vi "Process.vi"(8 "error in (no error)":errorcluster, 11 "RemoteControl":refnum<class "RemoteControl.lvclass">) -> (0 "error out":errorcluster, 3 "RemoteControl out":refnum<class "RemoteControl.lvclass">)   [LabVIEW 2019, in "RemoteControl.lvlib" / "RemoteControl.lvclass"]
doc: "---------------------------------------------------------------\nJKI State Machine Objects™\nhttp://jki.net/state-machine-objects/\nCopyright (C) 2005-2015, JKI <info@jki.net>\nALL RIGHTS RESERVED"
uses:
  RemoteControl.lvclass
  Typedefs/Message--Cluster.ctl
  Typedefs/RC Process Type--Enum.ctl
  <vilib>/ErrorRing/Error Ring.xnode
  <userlib>/LevyLab/Debug/Debug.lvlib
  C:/Program Files (x86)/National Instruments/LabVIEW 2019/vi.lib/JKI/JKI SMO/SMO/SMO.lvclass
  <vilib>/JKI/JKI SMO/SMO/SMO.lvclass
  <vilib>/JKI/JKI SMO/SMO/Typedefs/SMOState --Enum.ctl
  <vilib>/JKI/JKI SMO/SMO/Typedefs/Reserve State--Enum.ctl
  <vilib>/JKI/JKI SMO/SMO/Typedefs/Public Events.ctl
panel:
  out "Process Type":string
  out "Message Out":string
  out "Message In":string
  in  "delay response":bool
  in  "create server error":bool
  in  "create listener error":bool
  out "State History":string
  out "Connections":i32
  in  "Message Timing?":bool
  in  "timeout (ms) [500]":i32=500
  in  "stop":bool
  # "Remote Control"
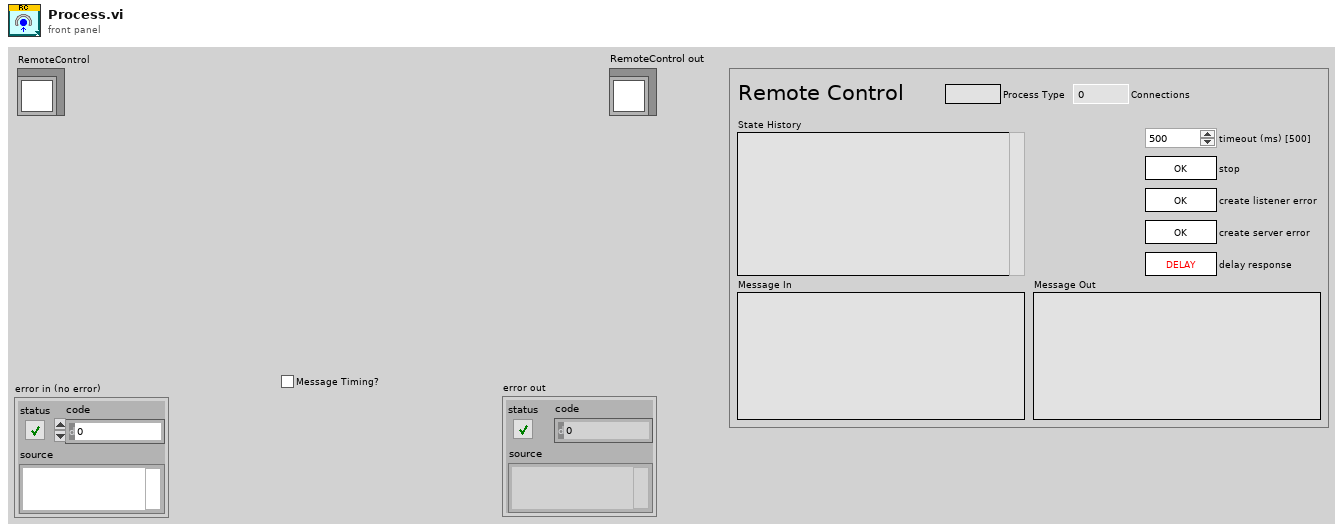
[diagram p1: front panel]
types:
  T1 = enum32{"invalid app kind", "Development System", "Run Time System", "Student Edition", "Embedded LabVIEW", "Evaluation", "Custom"}
  T2 = enum32{"Invalid", "Standard", "Closed", "Hidden", "Minimized", "Maximized"}
  T3 = typedef "RemoteControl.lvlib/RemoteControl.lvclass/Message--Cluster.ctl" = cluster{"Command":string, "Data":variant, "ID":string}
  T4 = typedef "RemoteControl.lvlib/RemoteControl.lvclass/RC Process Type--Enum.ctl" = enum16{"Listener", "Server", "Client"}
  T5 = typedef "RemoteControl.lvclass/Message--Cluster.ctl" = cluster{"Command":string, "Data":variant, "ID":string}
  T6 = typedef "RemoteControl.lvlib/RemoteControl.lvclass/PrivateEvents--RemoteControl.Configure.ctl" = cluster{"address":string, "Port":u16, "AllowedRemote":string, "Commands":string[], "timeout":i32}
  T7 = cluster{"Core":cluster{"Current VI Reference":refnum<vi>, "Close Panel on Exit?":bool, "Last Error":cluster{"error":errorcluster, "previous state":string, "remaining states":string}, "Shutdown?":bool}, "SelfRef":refnum<class "RemoteControl.lvclass">, "Listener":refnum<class "RemoteControl.lvclass">, "RC Process Type":T4, "Configure":T6, "Messages (in)":T3[], "Messages (out)":T3[], "state":enum16{"waiting", "processing"}, "to":i32}
  T8 = cluster{"Current VI Reference":refnum<vi>, "Close Panel on Exit?":bool, "Last Error":cluster{"error":errorcluster, "previous state":string, "remaining states":string}, "Shutdown?":bool}
  T9 = typedef "Debug.lvlib/Attribute.Debug.lvclass/DebugBehavior.ctl" = enum16{"Normal", "Debug"}
  T10 = typedef "SMO.lvclass/Public Events.ctl" = cluster{"Error":refnum<user-event>, "State":refnum<user-event>, "Reserve State":refnum<user-event>}
  T11 = typedef "SMO.lvclass/Protected Events.ctl" = cluster{"StopProcesses":refnum<user-event>, "AbortProcesses":refnum<user-event>, "Config Changed":refnum<user-event>, "Dependency":refnum<user-event>}
  T12 = typedef "RemoteControl.lvlib/RemoteControl.lvclass/PrivateEvents--Cluster.ctl" = cluster{"Configure":refnum<user-event>, "SendMessageToProcess":refnum<user-event>}
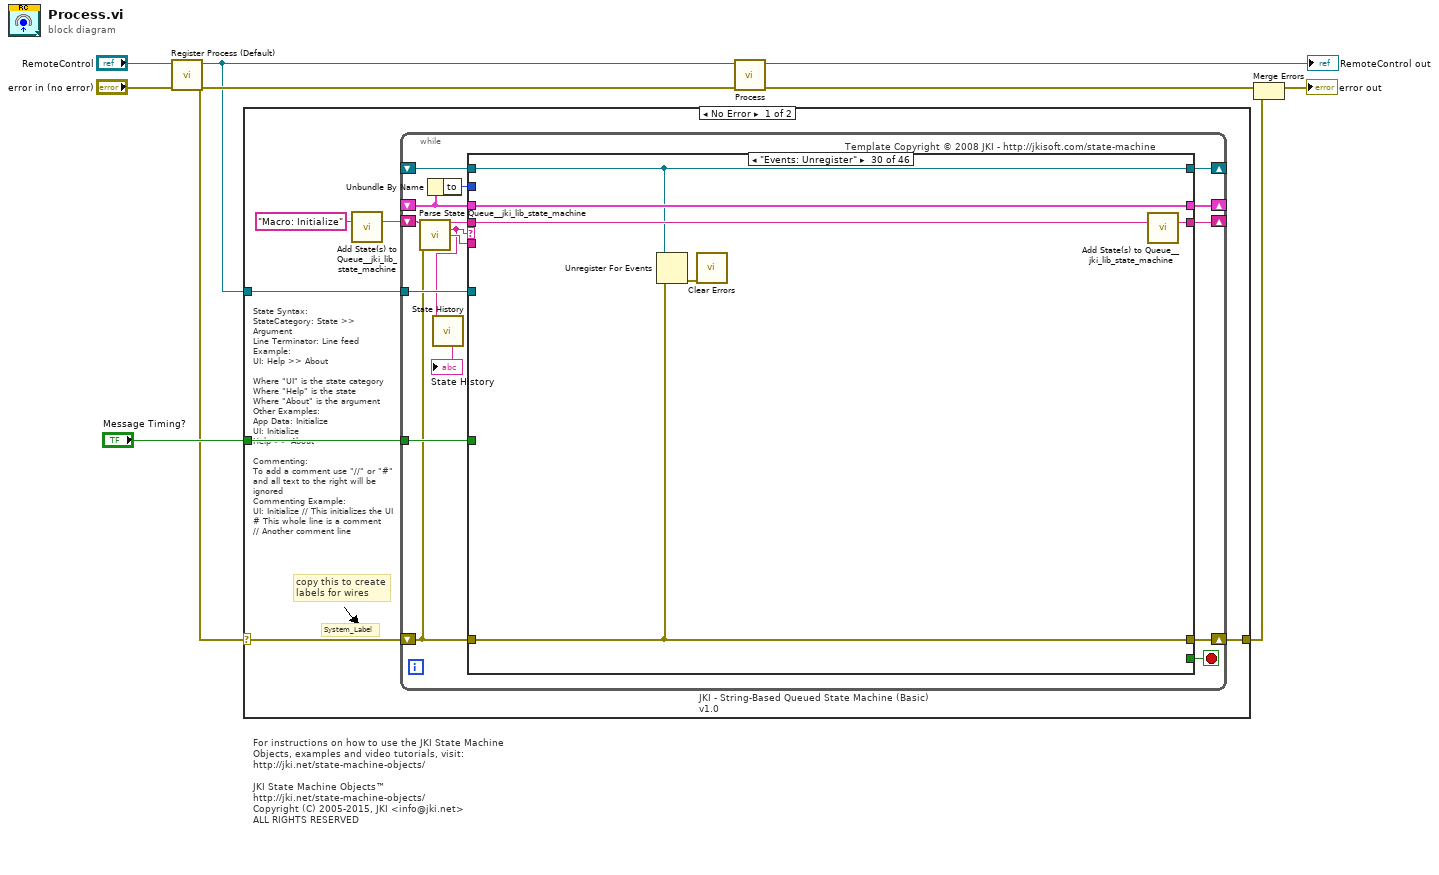
[diagram p0: block diagram]
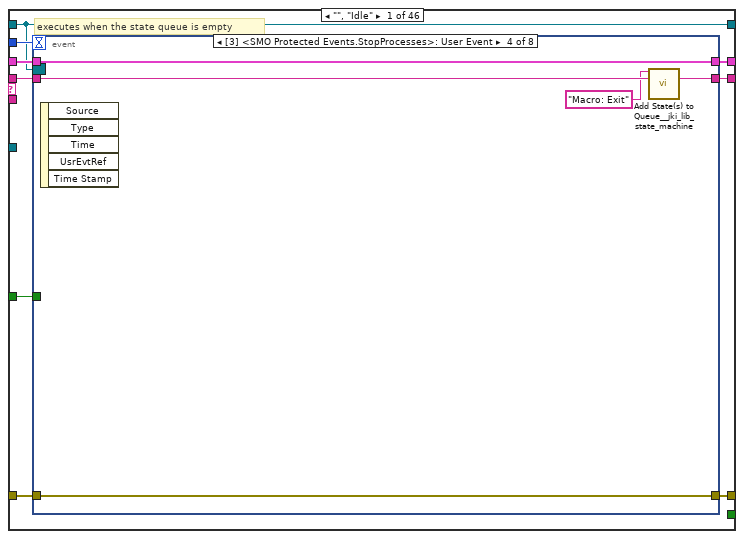
[diagram p2: hidden frame]
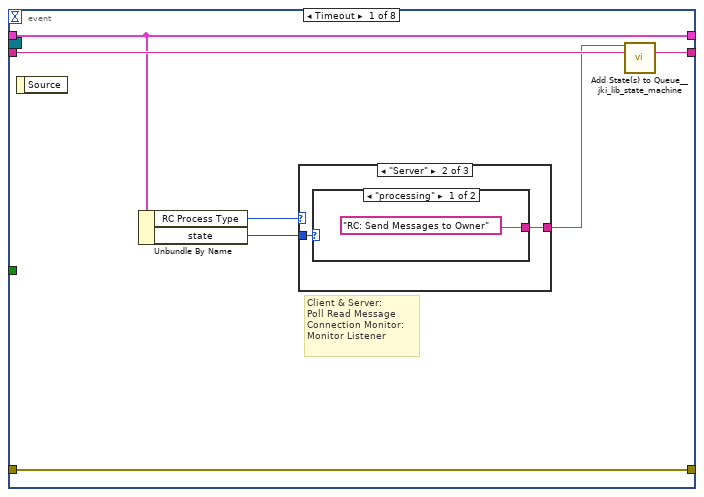
[diagram p3: hidden frame]
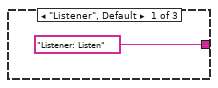
[diagram p4: hidden frame]
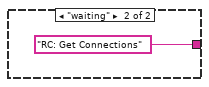
[diagram p5: hidden frame]
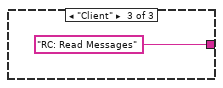
[diagram p6: hidden frame]
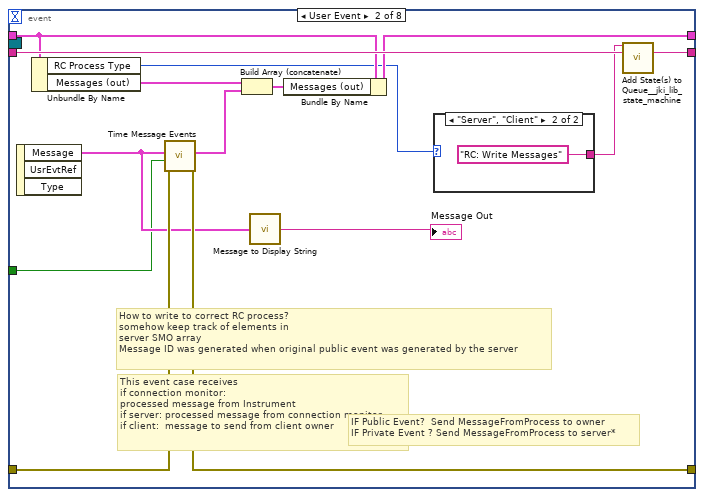
[diagram p7: hidden frame]
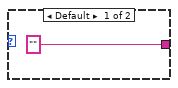
[diagram p8: hidden frame]
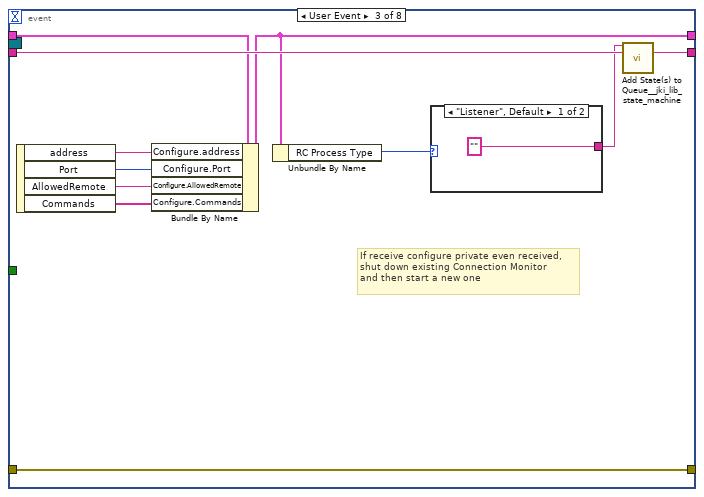
[diagram p9: hidden frame]
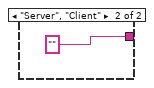
[diagram p10: hidden frame]
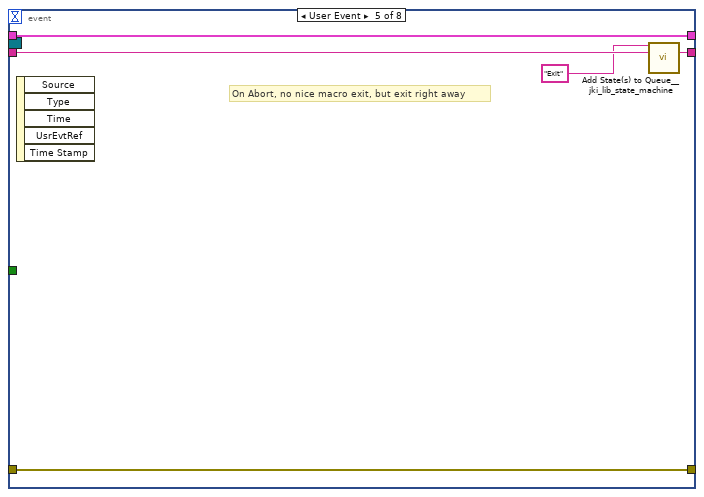
[diagram p11: hidden frame]
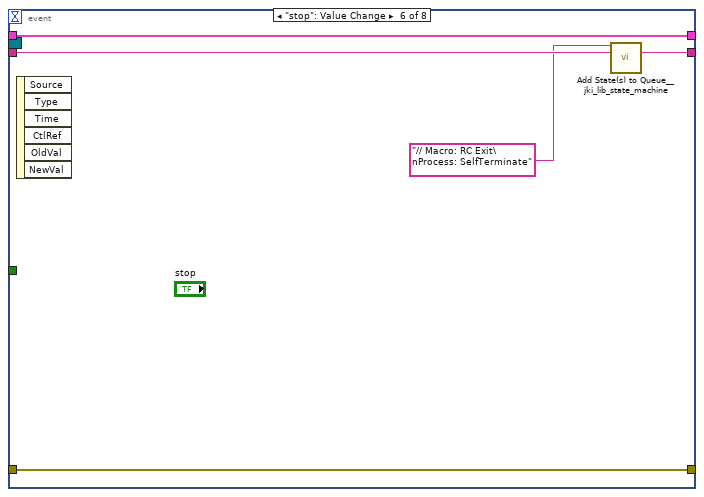
[diagram p12: hidden frame]
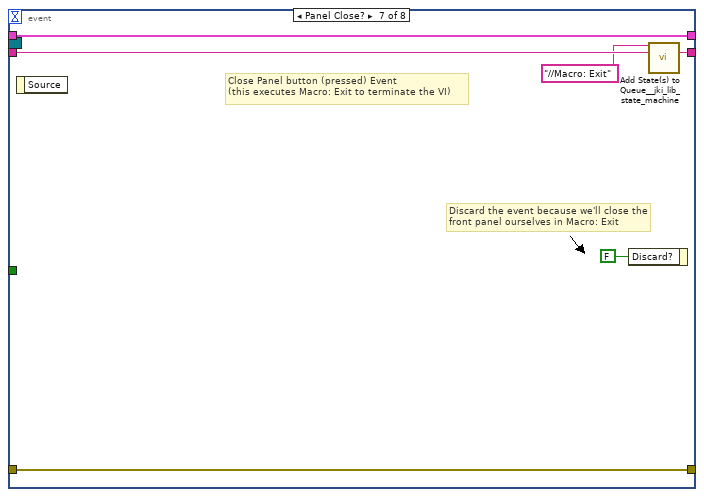
[diagram p13: hidden frame]
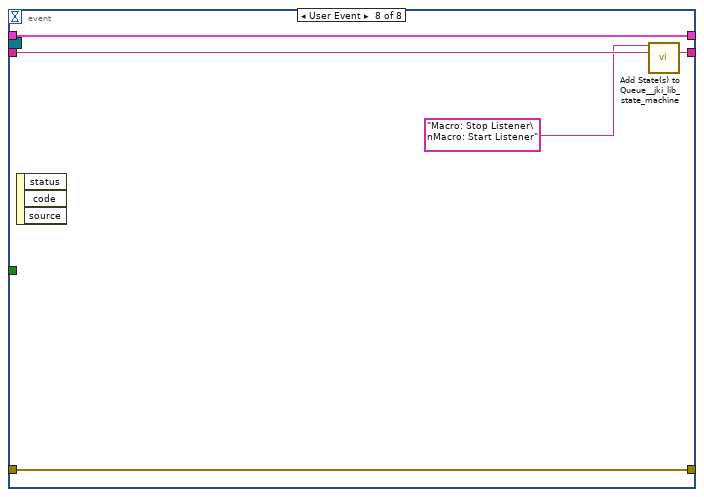
[diagram p14: hidden frame]
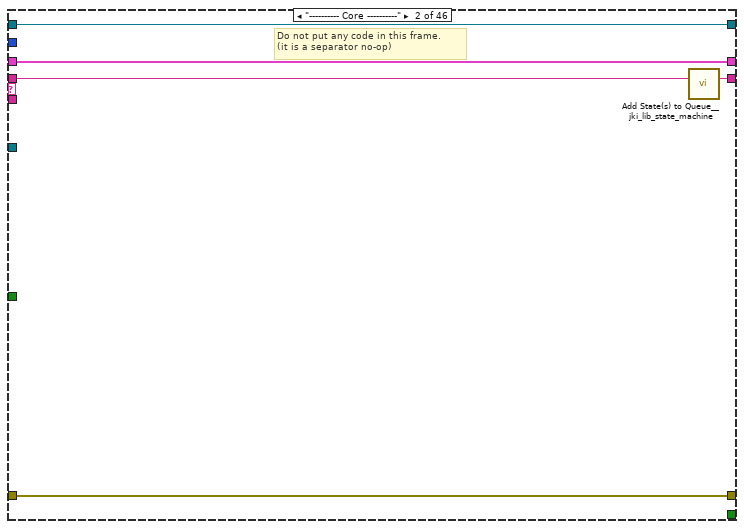
[diagram p15: hidden frame]
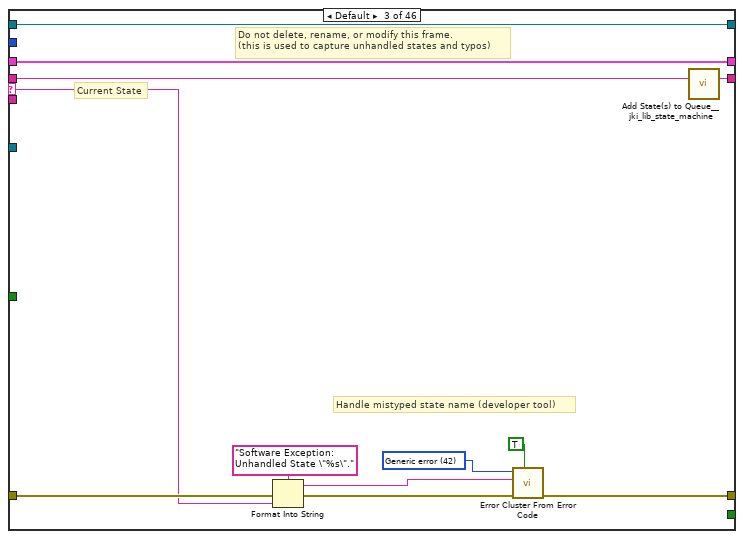
[diagram p16: hidden frame]
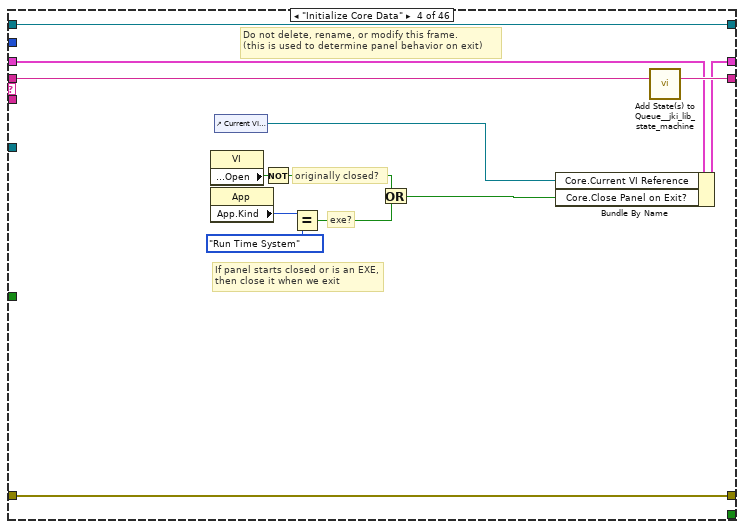
[diagram p17: hidden frame]
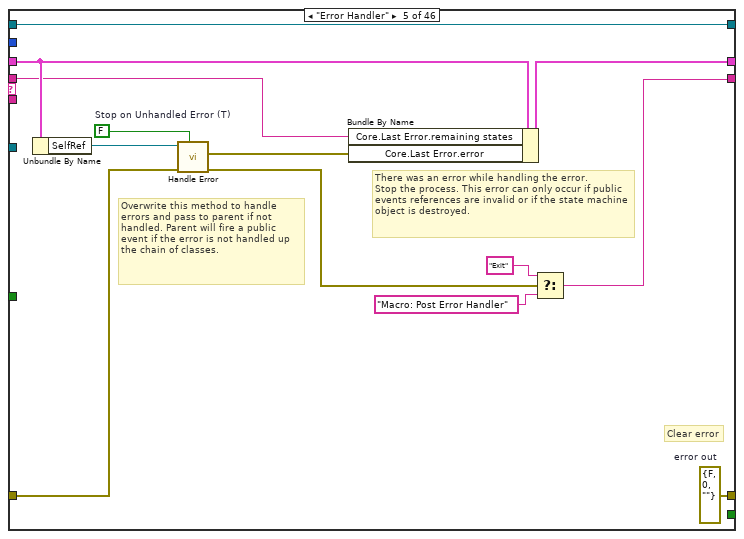
[diagram p18: hidden frame]
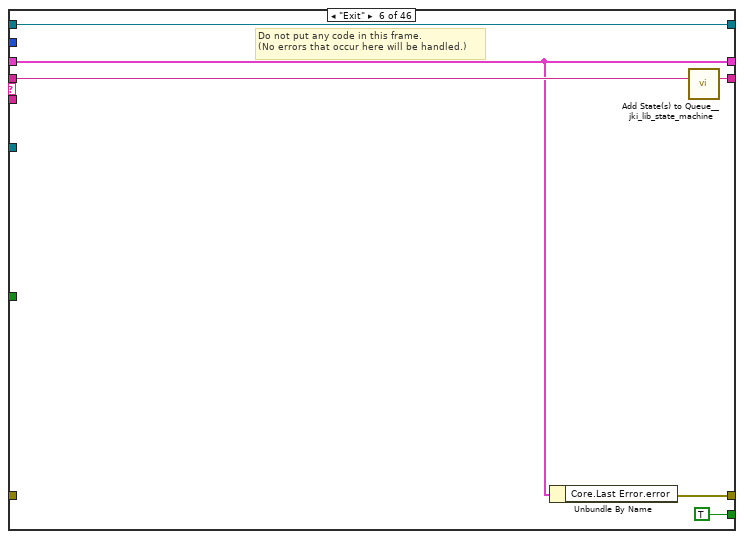
[diagram p19: hidden frame]
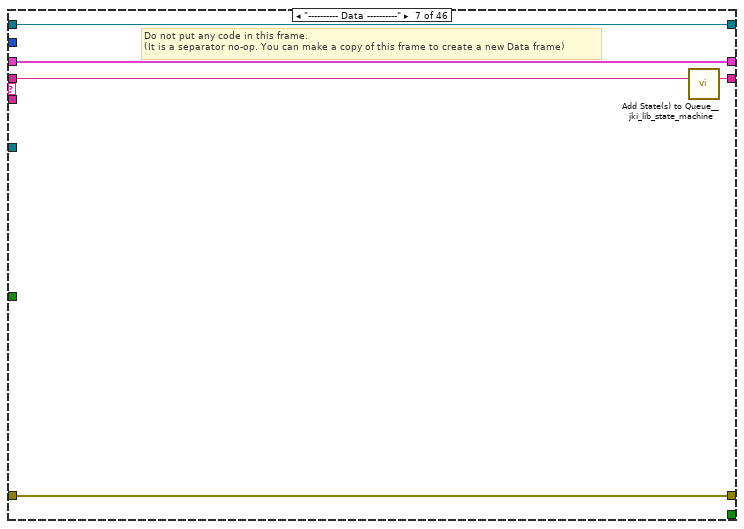
[diagram p20: hidden frame]
diagram:
  # "For instructions on how to use the JKI State Machine Objects, examples and video tutorials, visit:\nhttp://jki.net/state-machine-objects/\n\nJKI State Machine Objects™\nhttp://jki.net/state-machine-objects/\nCopyright (C) 2005-2015, JKI <info@jki.net>\nALL RIGHTS RESERVED"
  n1 = call <vilib>:"Register Process (Default).vi"("error in (no error)"="error in (no error)", "SMO"="RemoteControl") -> ("error out"=w3:errorcluster, "SelfRef"=w2:refnum<class "RemoteControl.lvclass">)  [unwired: 8 in]
  n2 = case shown="No Error" w3 {
    selector: w3 -> [w12 w662]
    tunnel: w2 -> [w13 _]
    tunnel: [w11 w662] -> w5
    tunnel: "Message Timing?" -> [w10 _]
    frame No Error {
      # "State Syntax:\nStateCategory: State >> Argument\nLine Terminator: Line feed\nExample:\nUI: Help >> About\n\nWhere \"UI\" is the state category\nWhere \"Help\" is the state\nWhere \"About\" is the argument\nOther Examples:\nApp Data: Initialize\nUI: Initialize\nHelp >> About\n\nCommenting:\nTo add a comment use \"//\" or \"#\" and all text to the right will be ignored\nCommenting Example:\nUI: Initialize // This initializes the UI\n# This whole line is a comment\n// Another comment line"
      # "copy this to create labels for wires"
      # "System_Label"
      n3 = call <vilib>:"Add State(s) to Queue__jki_lib_state_machine.vi"("State(s) in (\"\")"="Macro: Initialize") -> ("States Out"=w15:string)  [unwired: 14 in]
      n4 = while "JKI - String-Based Queued State Machine (Basic) v1.0" {
        shift-right: [w26] -> _
        shift-left: _ -> [w18]
        shift-right: [w28] -> w11
        shift-left: w12 -> [w21]
        shift-right: [w19] -> _
        shift-left: w15 -> [w29]
        tunnel: w13 -> [w25]
        shift-right: [w24] -> _
        shift-left: _ -> [w23]
        tunnel: w10 -> [w22]
        stop <- w27 stop-if-true
        # "Template Copyright © 2008 JKI - http://jkisoft.com/state-machine"
        n5 = call <vilib>:"Parse State Queue__jki_lib_state_machine.vi"("State Queue"=w29, "Error In (no error)"=w21) -> ("Remaining States"=w31:string, "Current State"=w20:string, "Arguments"=w30:string)  [unwired: 11 in]
        n6 = Unbundle By Name(w18) -> ("to"=w17:i32)
        n7 = call "State History.vi"("Current State"=w20) -> ("History"=→"State History":string)  [unwired: 10 in]
        n8 = case shown="\"Events: Unregister\"" w20 {
          selector: w20 -> [_ _ w115 _ _ _ _ _ _ _ _ _ _ _ _ _ _ _ _ _ _ _ _ _ _ _ _ _ _ _ _ _ _ _ _ _ _ _ _ _ _ _ _ _ _ _]
          tunnel: w31 -> [w40 w113 w119 w138 w141 w157 w162 w177 w184 w189 w199 w210 w226 w261 w266 w278 w293 w305 w317 w328 w337 w354 w376 w381 w392 w401 w406 w420 w434 w440 w445 w454 w475 w508 w542 w565 w578 w587 w596 w603 w614 w625 w630 w639 w651 w661]
          tunnel: w30 -> [_ _ _ _ _ _ _ _ _ _ _ w204 w221 w255 _ _ _ _ _ _ _ _ _ _ _ _ _ _ _ _ _ _ _ _ _ _ _ _ _ _ _ _ _ _ _ _]
          tunnel: [w37 w111 w121 w135 w150 w152 w160 w169 w181 w187 w191 w205 w219 w256 w264 w276 w284 w301 w309 w320 w335 w352 w374 w379 w384 w394 w404 w414 w429 w436 w441 w451 w463 w500 w535 w557 w573 w579 w588 w599 w609 w620 w626 w634 w640 w656] -> w28
          tunnel: [w39 w112 w118 w137 w144 w156 w161 w176 w183 w188 w198 w209 w225 w260 w265 w277 w292 w304 w316 w327 w336 w353 w375 w380 w391 w400 w405 w419 w433 w439 w444 w453 w474 w507 w541 w564 w577 w586 w595 w602 w613 w624 w629 w638 w650 w660] -> w19
          tunnel: [_ _ _ _ _ TRUE _ _ _ _ _ _ _ _ _ _ _ _ _ _ _ _ _ _ _ _ _ _ _ _ _ _ _ _ _ _ _ _ _ _ _ _ _ _ _ _] -> w27
          tunnel: [w35 w110 w117 w136 w148 w153 w159 w173 w180 w186 w196 w208 w223 w258 w263 w268 w282 w299 w313 w324 w332 w350 w365 w378 w389 w398 w403 w418 w432 w438 w443 w446 w472 w504 w533 w560 w574 w583 w590 w597 w606 w617 w628 w632 w647 w655] -> w26
          tunnel: w17 -> [w34 _ _ _ _ _ _ _ _ _ _ _ _ _ _ _ _ _ _ _ _ _ _ _ _ _ _ _ _ _ _ _ _ _ _ _ _ _ _ _ _ _ _ _ _ _]
          tunnel: w25 -> [_ _ _ _ _ _ _ w165 _ _ _ _ _ _ _ _ _ _ _ _ _ _ _ _ _ _ _ _ _ _ _ _ _ _ _ _ _ _ _ _ _ _ _ _ _ _]
          tunnel: [w33 w109 w114 w126 w151 w154 w158 w175 w179 w185 w197 w207 w220 w259 w262 w275 w291 w303 w315 w326 w334 w351 w370 w377 w390 w399 w402 w417 w431 w437 w442 w452 w473 w506 w540 w563 w576 w585 w594 w601 w612 w623 w627 w637 w649 w659] -> w24
          tunnel: w23 -> [w33 w109 w114 w126 w151 w154 w158 w175 w179 w185 w197 w207 w220 w259 w262 w275 w291 w303 w315 w326 w334 w351 w370 w377 w390 w399 w402 _ w427 w437 w442 w452 w473 w506 w540 w563 w576 w585 w594 w601 w612 w623 w627 w637 w649 w659]
          tunnel: w22 -> [w32 _ _ _ _ _ _ _ _ _ _ _ _ _ _ _ _ _ _ _ _ _ _ _ _ _ _ _ _ _ _ w449 _ w505 w538 _ _ _ _ _ _ _ _ _ _ _]
          tunnel: w21 -> [w36 w111 w120 w135 w146 _ w160 w169 w182 w187 w190 w206 w224 w257 w264 w276 w283 w301 w310 w321 w335 w352 w374 w379 w385 w395 w404 w415 w430 w436 w441 w448 w469 w490 w536 w558 w566 w580 w589 w600 w610 w621 w626 w635 w644 w657]
          tunnel: w18 -> [w38 w110 w117 w129 w149 w153 w159 _ w180 w186 w196 w208 w223 w258 w263 w268 w281 w299 w313 w324 w332 w347 w364 w378 w389 w393 w403 w418 w432 w438 w443 w446 w471 w492 w534 w561 w575 w584 w591 w597 w607 w618 w628 w631 w648 w655]
          frame "", "Idle" {
            # "executes when the state queue is empty"
            n9 = event shown="[3] <SMO Protected Events.StopProcesses>: User Event" {
              selector: w33 -> [_ _ _ _ _ _ _ _]
              dyn-events: _ -> [_ _ _ _ _ _ _ _]
              timeout: w34 -> [_ _ _ _ _ _ _ _]
              tunnel: w40 -> [w47 w67 w79 w87 w92 w96 w103 w108]
              tunnel: [w46 w66 w78 w86 w91 w97 w102 w107] -> w39
              tunnel: w38 -> [w42 w63 w77 w84 w89 w95 w100 w105]
              tunnel: [w45 w60 w80 w85 w90 w93 w101 w106] -> w37
              tunnel: w36 -> [w45 w59 w80 w85 w90 w93 w101 w106]
              tunnel: [w42 w65 w75 w84 w89 w95 w100 w105] -> w35
              tunnel: w32 -> [_ w54 _ _ _ _ _ _]
              event Timeout {
                # "Client & Server:\nPoll Read Message\nConnection Monitor:\nMonitor Listener"
                n10 = event-data() -> ()  [unwired: 1 in, 1 out]
                n11 = Unbundle By Name(w42) -> ("RC Process Type"=w43:T4, "state"=w41:enum16{"waiting", "processing"})
                n12 = case shown="\"Server\"" w43 {
                  tunnel: ["Listener: Listen" ("State(s) in Front (\"\")") w50 "RC: Read Messages" ("State(s) in Front (\"\")")] -> w44
                  tunnel: w41 -> [_ w49 _]
                  frame "Listener", Default {
                  }
                  frame "Server" {
                    n13 = case shown="\"processing\"" w49 {
                      tunnel: ["RC: Send Messages to Owner" ("State(s) in Front (\"\")") "RC: Get Connections" ("State(s) in Front (\"\")")] -> w50
                      frame "processing" {
                      }
                      frame "waiting" {
                      }
                    }
                  }
                  frame "Client" {
                  }
                }
                n14 = call <vilib>:"Add State(s) to Queue__jki_lib_state_machine.vi"("State(s) in Front (\"\")"=w44, "State(s) in (\"\")"=w47) -> ("States Out"=w46:string)  [unwired: 13 in]
              }
              event User Event {
                # "IF Public Event?  Send MessageFromProcess to owner\nIF Private Event ? Send MessageFromProcess to server*"
                # "How to write to correct RC process?\nsomehow keep track of elements in\nserver SMO array\nMessage ID was generated when original public event was generated by the server"
                # "This event case receives\nif connection monitor:\nprocessed message from Instrument\nif server: processed message from connection monitor\nif client:  message to send from client owner"
                n15 = event-data() -> ("Message"=w56:T5)  [unwired: 1 in, 2 out]
                n16 = Unbundle By Name(w63) -> ("RC Process Type"=w58:T4, "Messages (out)"=w62:T3[])
                n17 = call "Time Message Events.vi"("error in (no error)"=w59, "Debug Mode"=w54, "Message in"=w56) -> ("error out"=w60:errorcluster, "Message out"=w57:T3)  [unwired: 5 in, 2 out]
                n18 = Build Array (concatenate)(w62, w57) -> (w61:T3[])
                n19 = call "Message to Display String.vi"("Message"=w56) -> ("message string"=→"Message Out":string)
                n20 = Bundle By Name(cluster=w63, "Messages (out)"=w61) -> (w65:T7)
                n21 = case shown="\"Server\", \"Client\"" w58 {
                  tunnel: ["" ("State(s) in Front (\"\")") "RC: Write Messages" ("State(s) in Front (\"\")")] -> w64
                  frame Default {
                  }
                  frame "Server", "Client" {
                  }
                }
                n22 = call <vilib>:"Add State(s) to Queue__jki_lib_state_machine.vi"("State(s) in Front (\"\")"=w64, "State(s) in (\"\")"=w67) -> ("States Out"=w66:string)  [unwired: 13 in]
              }
              event User Event {
                # "If receive configure private even received,\nshut down existing Connection Monitor \nand then start a new one"
                n23 = event-data() -> ("address"=w70:string, "Port"=w71:u16, "AllowedRemote"=w72:string, "Commands"=w73:string[])  [unwired: 1 in]
                n24 = Bundle By Name(cluster=w77, "Configure.address"=w70, "Configure.Port"=w71, "Configure.AllowedRemote"=w72, "Configure.Commands"=w73) -> (w75:T7)
                n25 = Unbundle By Name(w75) -> ("RC Process Type"=w76:T4)
                n26 = case shown="\"Listener\", Default" w76 {
                  tunnel: ["" ("State(s) in Front (\"\")") "" ("State(s) in Front (\"\")")] -> w74
                  frame "Listener", Default {
                  }
                  frame "Server", "Client" {
                  }
                }
                n27 = call <vilib>:"Add State(s) to Queue__jki_lib_state_machine.vi"("State(s) in Front (\"\")"=w74, "State(s) in (\"\")"=w79) -> ("States Out"=w78:string)  [unwired: 13 in]
              }
              event User Event {
                n28 = event-data() -> ()  [unwired: 1 in, 5 out]
                n29 = call <vilib>:"Add State(s) to Queue__jki_lib_state_machine.vi"("State(s) in Front (\"\")"="Macro: Exit", "State(s) in (\"\")"=w87) -> ("States Out"=w86:string)  [unwired: 13 in]
              }
              event User Event {
                # "On Abort, no nice macro exit, but exit right away"
                n30 = event-data() -> ()  [unwired: 1 in, 5 out]
                n31 = call <vilib>:"Add State(s) to Queue__jki_lib_state_machine.vi"("State(s) in Front (\"\")"="Exit", "State(s) in (\"\")"=w92) -> ("States Out"=w91:string)  [unwired: 13 in]
              }
              event "stop": Value Change {
                n32 = event-data() -> ()  [unwired: 1 in, 6 out]
                n33 = call <vilib>:"Add State(s) to Queue__jki_lib_state_machine.vi"("State(s) in Front (\"\")"="// Macro: RC Exit\nProcess: SelfTerminate" ("State(s) in Front (\"\")"), "State(s) in (\"\")"=w96) -> ("States Out"=w97:string)  [unwired: 13 in]
              }
              event Panel Close? {
                # "Discard the event because we'll close the front panel ourselves in Macro: Exit"
                # "Close Panel button (pressed) Event\n(this executes Macro: Exit to terminate the VI)"
                n34 = event-data() -> ()  [unwired: 1 in, 1 out]
                n35 = event-data("Discard?"=FALSE) -> ()  [unwired: 1 in, 1 out]
                n36 = call <vilib>:"Add State(s) to Queue__jki_lib_state_machine.vi"("State(s) in Front (\"\")"="//Macro: Exit", "State(s) in (\"\")"=w103) -> ("States Out"=w102:string)  [unwired: 13 in]
              }
              event User Event {
                n37 = event-data() -> ()  [unwired: 1 in, 3 out]
                n38 = call <vilib>:"Add State(s) to Queue__jki_lib_state_machine.vi"("State(s) in Front (\"\")"="Macro: Stop Listener\nMacro: Start Listener", "State(s) in (\"\")"=w108) -> ("States Out"=w107:string)  [unwired: 13 in]
              }
            }
          }
          frame "---------- Core ----------" {
            # "Do not put any code in this frame.\n(it is a separator no-op)"
            n39 = call <vilib>:"Add State(s) to Queue__jki_lib_state_machine.vi"("State(s) in (\"\")"=w113) -> ("States Out"=w112:string)  [unwired: 14 in]
          }
          frame Default {
            w124 = 42 items=["No error", "Argument error", "Memory is full", "Out of zone", "End of file", "File already open", "Generic file I/O error", "File not found", "File permission error", "Disk is full", "Duplicate path", "Too many files open", "System feature not enabled", "Resource file not found", "Cannot add resource", "Resource not found", "Image not found", "Image memory error", "Pen does not exist", "Config type invalid", "Config token not found", "Config parse error", "Config memory error", "Bad external code format", "Bad external code offset", "External code not present", "Null window", "Destroy window error", "Null menu", "Print aborted", "Bad print record", "Print driver error", "Windows error during printing", "Memory error during printing", "Print dialog error", "Generic print error", "Invalid device refnum", "Device not found", "Device parameter error", "Device unit error", "Cannot open device", "Device call aborted", "Generic error", "Cancelled by user", "Object ID too low", "Object ID too high", "Object not in heap", "Unknown heap", "Unknown object (invalid DefProc)", "Unknown object (DefProc not in table)", "Message out of range", "Invalid (null) method", "Unknown message", "Manager call not supported", "Bad address", "Network operation in progress", "Network operation timed out", "Connection is busy", "Network attribute not supported", "Network error", "Address in use", "System out of memory", "Connection aborted", "Connection refused", "Not connected", "Already connected", "Connection closed", "Initialization error (interapplication manager)", "Bad occurrence", "Wait on unbound occurrence handler", "Occurrence queue overflow", "Datalog type conflict", "Unused", "Unrecognized type (interapplication manager)", "Memory corrupt", "Failed to make temporary DLL", "Old CIN version", "Drag socket not found", "Failed to load drop-object", "Failed to register OLE object", "Failed to release OLE object", "Format specifier type mismatch", "Unknown format specifier", "Too few format specifiers", "Too many format specifiers", "Scan failed", "Newer CIN version", "Error converting to variant", "Runtime menu error", "Password tampered", "Variant attribute not found", "Incompatible variant data type", "Event data is not available", "Event Store is not present", "Occurrence is not found", "Event Queue is not created", "Event info is not available", "Refnum passed is NULL", "Error retrieving Class GUID", "Error retrieving CoClass GUID", "Error retrieving TypeLib GUID.", "Bad built application magic bytes.", "Specific driver is different from the specific driver associated with the Logical Name.", "There is no session opened to the class driver.", "Max Error", "MAX - Error with config objects", "MAX - Error loading configuration", "MAX - Group not supported"]
            # "Current State"
            # "Do not delete, rename, or modify this frame.\n(this is used to capture unhandled states and typos)"
            # "Handle mistyped state name (developer tool)"
            n40 = Format Into String(format string="Software Exception: Unhandled State \"%s\"." ("message"), error in=w120, w115) -> (resulting string=w123:string, error out=w122:errorcluster)  [unwired: 1 in]
            n41 = call <vilib>:"Error Cluster From Error Code.vi"("show call chain? (False)"=TRUE, "error in (no error)"=w122, "error message (\"\")"=w123, "error code (0)"=w124) -> ("error out"=w121:errorcluster)  [unwired: 5 in]
            n42 = call <vilib>:"Add State(s) to Queue__jki_lib_state_machine.vi"("State(s) in (\"\")"=w119) -> ("States Out"=w118:string)  [unwired: 14 in]
          }
          frame "Initialize Core Data" {
            # "Do not delete, rename, or modify this frame.\n(this is used to determine panel behavior on exit)"
            # "originally closed?"
            # "exe?"
            # "If panel starts closed or is an EXE, then close it when we exit"
            n43 = property class="VI"() -> ("Front Panel.Open"=w134:bool)  [unwired: 2 in, 2 out]
            n44 = property class="App"() -> ("App.Kind"=w133:T1)  [unwired: 2 in, 2 out]
            n45 = control-ref of="Current VI Reference"() -> (w127:refnum<vi>)
            n46 = Not(x=w134) -> (.not. x?=w131:bool)
            n47 = Equal?(x=w133, y=T1."Run Time System" ("Application:Kind")) -> (x = y?=w130:bool)
            n48 = Or(x=w131, y=w130) -> (x .or. y?=w128:bool)
            n49 = Bundle By Name(cluster=w129, "Core.Current VI Reference"=w127, "Core.Close Panel on Exit?"=w128) -> (w136:T7)
            n50 = call <vilib>:"Add State(s) to Queue__jki_lib_state_machine.vi"("State(s) in (\"\")"=w138) -> ("States Out"=w137:string)  [unwired: 14 in]
          }
          frame "Error Handler" {
            w147 = FALSE  # Stop on Unhandled Error (T)
            w150 = errorcluster {"status"=FALSE, "code"=0, "source"=""}  # error out
            # "There was an error while handling the error.\nStop the process. This error can only occur if public events references are invalid or if the state machine object is destroyed."
            # "Clear error"
            # "Overwrite this method to handle errors and pass to parent if not handled. Parent will fire a public event if the error is not handled up the chain of classes."
            n51 = Unbundle By Name(w149) -> ("SelfRef"=w145:refnum<class "RemoteControl.lvclass">)
            n52 = call-dynamic "Handle Error.vi"("Stop on Unhandled Error (T)"=w147, "error in"=w146, "SMO"=w145) -> ("handling error"=w142:errorcluster, "Unhandled error"=w143:errorcluster)  [unwired: 6 in, 1 out]
            n53 = Bundle By Name(cluster=w149, "Core.Last Error.remaining states"=w141, "Core.Last Error.error"=w143) -> (w148:T7)
            n54 = Select(t="Exit", s=w142, f="Macro: Post Error Handler") -> (s? t:f=w144:string)
          }
          frame "Exit" {
            # "Do not put any code in this frame.\n(No errors that occur here will be handled.)"
            n55 = Unbundle By Name(w153) -> ("Core.Last Error.error"=w152:errorcluster)
            n56 = call <vilib>:"Add State(s) to Queue__jki_lib_state_machine.vi"("State(s) in (\"\")"=w157) -> ("States Out"=w156:string)  [unwired: 14 in]
          }
          frame "---------- Data ----------" {
            # "Do not put any code in this frame.\n(It is a separator no-op. You can make a copy of this frame to create a new Data frame)"
            n57 = call <vilib>:"Add State(s) to Queue__jki_lib_state_machine.vi"("State(s) in (\"\")"=w162) -> ("States Out"=w161:string)  [unwired: 14 in]
          }
          frame "Data: Initialize" {
            w166 = 10  # to
            w167 = enum16{"waiting", "processing"}."waiting"  # state
            w168 = refnum<class "RemoteControl.lvclass"> refnum  # Listener
            w170 = T3[] []  # Messages (out)
            w171 = T3[] []  # Messages (in)
            w174 = T8 {"Current VI Reference"=refnum, "Close Panel on Exit?"=FALSE, "Last Error"={"error"={"status"=FALSE, "code"=0, "source"=""}, "previous state"="", "remaining states"=""}, "Shutdown?"=FALSE}  # Core
            # "do not delete - used by framework"
            # "Initialize the shift-register data, here.\n(data names are defined by what you wire into the bundle function)"
            n58 = Unbundle By Name(w165) -> ("RC Process Type"=w163:T4, "Configure"=w172:T6)
            n59 = Format Into String(w163) -> (resulting string=→"Process Type":string)  [unwired: 3 in, 1 out]
            n60 = Bundle("Core"=w174, "SelfRef"=w165, "Listener"=w168, "RC Process Type"=w163, "Configure"=w172, "Messages (in)"=w171, "Messages (out)"=w170, "state"=w167, "to"=w166) -> (w173:T7)  [unwired: 1 in]
            n61 = call <vilib>:"Add State(s) to Queue__jki_lib_state_machine.vi"("State(s) in (\"\")"=w177) -> ("States Out"=w176:string)  [unwired: 14 in]
          }
          frame "Data: Cleanup" {
            # "Cleanup any data and references, here.\n(this is called automatically, by the Macro: Exit)"
            n62 = Unbundle By Name(w180) -> ("Core.Current VI Reference"=w178:refnum<vi>)
            n63 = Close Reference(reference=w178, error in (no error)=w182) -> (error out=w181:errorcluster)
            n64 = call <vilib>:"Add State(s) to Queue__jki_lib_state_machine.vi"("State(s) in (\"\")"=w184) -> ("States Out"=w183:string)  [unwired: 14 in]
          }
          frame "---------- UI ----------" {
            # "Do not put any code in this frame.\n(It is a separator no-op. You can make a copy of this frame to create a new UI frame)"
            n65 = call <vilib>:"Add State(s) to Queue__jki_lib_state_machine.vi"("State(s) in (\"\")"=w189) -> ("States Out"=w188:string)  [unwired: 14 in]
          }
          frame "UI: Initialize" {
            # "Initialize the User Interface, here.\n(this is called automatically, by the Macro: Init)"
            n66 = Unbundle By Name(w196) -> ("RC Process Type"=w195:T4)
            n67 = case shown="\"Server\", Default" w195 {
              tunnel: [FALSE TRUE] -> w194
              tunnel: [TRUE FALSE] -> w193
              frame "Listener" {
              }
              frame "Server", Default {
              }
            }
            n68 = call <userlib>:"Fit VI window to Largest Dec__ogtk.vi"("error in (no error)"=w190, "border spacing (2 px)"=0) -> ("error out"=w191:errorcluster)  [unwired: 4 in, 1 out]
            n69 = property on="create server error" class="Bool (strict)"("Visible"=w194) -> ()  [unwired: 2 in, 2 out]
            n70 = property on="create listener error" class="Bool (strict)"("Visible"=w193) -> ()  [unwired: 2 in, 2 out]
            n71 = call <vilib>:"Add State(s) to Queue__jki_lib_state_machine.vi"("State(s) in (\"\")"=w199) -> ("States Out"=w198:string)  [unwired: 14 in]
          }
          frame "UI: Cursor Set" {
            # "Argument"
            # "Initialize the User Interface, here.\n(this is called automatically, by the Macro: Init)"
            n72 = disable-structure shown="Default" {
              disable-tunnel: w206 -> [w211 w214]
              disable-tunnel: [w211 w213] -> w205
              disable-tunnel: w204 -> [_ w212]
              frame condition #0 {
              }
              frame condition #1 (active) {
                n73 = case shown="\"Idle\", Default" w212 {
                  tunnel: w214 -> [w216 w218]
                  tunnel: [w215 w217] -> w213
                  frame "Idle", Default {
                    n74 = call <vilib>:"Unset Busy.vi"("error in (no error)"=w216) -> ("error out"=w215:errorcluster)  [unwired: 10 in]
                  }
                  frame "Busy" {
                    n75 = call <vilib>:"Set Busy.vi"("error in (no error)"=w218) -> ("error out"=w217:errorcluster)  [unwired: 9 in, 1 out]
                  }
                }
              }
            }
            n76 = call <vilib>:"Add State(s) to Queue__jki_lib_state_machine.vi"("State(s) in (\"\")"=w210) -> ("States Out"=w209:string)  [unwired: 14 in]
          }
          frame "UI: Front Panel State" {
            # "Argument"
            # "Set Front Panel Open or Closed\n(Usage: \"UI: Front Panel State >> Open|Close\")"
            n77 = Unbundle By Name(w223) -> ("Core.Current VI Reference"=w222:refnum<vi>)
            n78 = disable-structure shown="Default" {
              disable-tunnel: w224 -> [w230 w251]
              disable-tunnel: [w229 w251] -> w219
              disable-tunnel: w222 -> [w228 _]
              disable-tunnel: w221 -> [w227 _]
              frame condition #0 (active) {
                n79 = case shown="\"Close\"" w227 {
                  tunnel: w230 -> [w234 w245]
                  tunnel: [w235 w246] -> w229
                  tunnel: w228 -> [_ _]
                  frame "Open", Default {
                    n80 = property class="VI"(error in=w234) -> (reference out=w232:refnum<vi>, error out=w233:errorcluster, "FP.State"=w231:T2)  [unwired: 1 in]
                    n81 = case shown="\"Closed\"" w231 {
                      tunnel: [w238 w241] -> w235
                      tunnel: w233 -> [w237 w241]
                      tunnel: w232 -> [w236 _]
                      frame "Closed" {
                        n82 = invoke class="VI" method="FP.Open"(reference=w236, error in=w237, "Activate"=TRUE, "State"=T2."Standard") -> (error out=w238:errorcluster)  [unwired: 1 in, 4 out]
                      }
                      frame Default {
                      }
                    }
                  }
                  frame "Close" {
                    n83 = property class="VI"(error in=w245) -> (reference out=w243:refnum<vi>, error out=w244:errorcluster, "FP.State"=w242:T2)  [unwired: 1 in]
                    n84 = case shown="Default" w242 {
                      tunnel: [w247 w250] -> w246
                      tunnel: w244 -> [w247 w249]
                      tunnel: w243 -> [_ w248]
                      frame "Invalid", "Closed" {
                      }
                      frame Default {
                        n85 = invoke class="VI" method="FP.Close"(reference=w248, error in=w249) -> (error out=w250:errorcluster)  [unwired: 1 in, 2 out]
                      }
                    }
                  }
                }
              }
              frame condition #1 {
              }
            }
            n86 = call <vilib>:"Add State(s) to Queue__jki_lib_state_machine.vi"("State(s) in (\"\")"=w226) -> ("States Out"=w225:string)  [unwired: 14 in]
          }
          frame "UI: Wait" {
            n87 = Scan From String(format string="%d", input string=w255, default 1=u32 0 ("default value 1")) -> (output 1=w253:u32)  [unwired: 2 in, 3 out]
            n88 = call <userlib>:"Wait (ms)__ogtk.vi"("error in (no error)"=w257, "milliseconds to wait"=w253) -> ("error out"=w256:errorcluster)  [unwired: 8 in, 1 out]
            n89 = call <vilib>:"Add State(s) to Queue__jki_lib_state_machine.vi"("State(s) in (\"\")"=w261) -> ("States Out"=w260:string)  [unwired: 14 in]
          }
          frame "---------- Macro ----------" {
            # "Do not put any code in this frame.\n(It is a separator no-op. You can make a copy of this frame to create a new Macro frame)"
            n90 = call <vilib>:"Add State(s) to Queue__jki_lib_state_machine.vi"("State(s) in (\"\")"=w266) -> ("States Out"=w265:string)  [unwired: 14 in]
          }
          frame "Macro: Initialize" {
            # "Initialization Macro\n(This is called once, when the VI starts)"
            n91 = call <vilib>:"Add State(s) to Queue__jki_lib_state_machine.vi"("State(s) in Front (\"\")"="UI: Initialize", "State(s) in (\"\")"="UI: Front Panel State >> Close", "State(s) at Back (\"\")"="Macro: Debug\nMacro: RC Initialize") -> ("States Out"=w269:string)  [unwired: 12 in]
            n92 = call <vilib>:"Add State(s) to Queue__jki_lib_state_machine.vi"("State(s) in Front (\"\")"="Data: Initialize\nInitialize Core Data\nEvents: Register", "State(s) in (\"\")"="Process: Sync", "State(s) at Back (\"\")"=w269) -> ("States Out"=w273:string)  [unwired: 12 in]
            n93 = call <vilib>:"Add State(s) to Queue__jki_lib_state_machine.vi"("State(s) in Front (\"\")"=w273, "State(s) in (\"\")"=w278) -> ("States Out"=w277:string)  [unwired: 13 in]
          }
          frame "Macro: Debug" {
            # "exe?"
            # "If pane is an EXE, then close it when we exit"
            # "Macro: Debug\n(get debug behavior, determine UI and determine shutdown behavior)"
            n94 = Unbundle By Name(w281) -> ("Core.Close Panel on Exit?"=w285:bool, "SelfRef"=w290:refnum<class "RemoteControl.lvclass">)
            n95 = property class="App"() -> ("App.Kind"=w288:T1)  [unwired: 2 in, 2 out]
            n96 = Equal?(x=w288, y=T1."Run Time System" ("Application:Kind")) -> (x = y?=w280:bool)
            n97 = call <userlib>:"Get Debug Mode.vi"("error in (no error)"=w283, "SMO"=w290) -> ("error out"=w284:errorcluster, "Behavior"=w289:T9)  [unwired: 7 in, 1 out]
            n98 = case shown="\"Debug\"" w289 {
              tunnel: [_ "UI: Front Panel State >> Open\nUI: Wait >> 1000"] -> w279
              tunnel: [w294 w295] -> w286
              tunnel: w285 -> [w294 _]
              tunnel: w280 -> [_ w297]
              frame "Normal", Default {
                # "respect core.close"
              }
              frame "Debug" {
                # "keep panel open\nunless exe"
                n99 = Or(x=w297, y=FALSE) -> (x .or. y?=w295:bool)
              }
            }
            n100 = Bundle By Name(cluster=w281, "Core.Close Panel on Exit?"=w286) -> (w282:T7)
            n101 = call <vilib>:"Add State(s) to Queue__jki_lib_state_machine.vi"("State(s) in Front (\"\")"=w279, "State(s) in (\"\")"=w293) -> ("States Out"=w292:string)  [unwired: 13 in]
          }
          frame "Macro: RC Initialize" {
            n102 = Unbundle By Name(w299) -> ("RC Process Type"=w302:T4)
            n103 = case shown="\"Server\"" w302 {
              tunnel: ["Listener: Start Listener" ("State(s) in Front (\"\")") "Macro: Start Listener\nRC: Open Server Connection" ("State(s) in Front (\"\")") "RC: Open Client Connection" ("State(s) in Front (\"\")")] -> w300
              frame "Listener", Default {
              }
              frame "Server" {
              }
              frame "Client" {
              }
            }
            n104 = call <vilib>:"Add State(s) to Queue__jki_lib_state_machine.vi"("State(s) in Front (\"\")"=w300, "State(s) in (\"\")"=w305) -> ("States Out"=w304:string)  [unwired: 13 in]
          }
          frame "Macro: Start Listener" {
            n105 = Unbundle By Name(w313) -> ("SelfRef"=w312:refnum<class "RemoteControl.lvclass">)
            n106 = call <vilib>:"Get LV Class Name.vi"("error in (no error)"=w310, "object"=w312) -> ("error out"=w309:errorcluster, "class name"=w311:string)  [unwired: 8 in]
            n107 = case shown="\"RemoteControl.STM.lvclass\"" w311 {
              tunnel: ["" ("State(s) in Front (\"\")") "RC: Create Listener SMO\nEvents: Register Listener SMO\nRC: Start Listener SMO" ("State(s) in Front (\"\")")] -> w314
              frame Default {
              }
              frame "RemoteControl.STM.lvclass" {
              }
            }
            n108 = call <vilib>:"Add State(s) to Queue__jki_lib_state_machine.vi"("State(s) in Front (\"\")"=w314, "State(s) in (\"\")"=w317) -> ("States Out"=w316:string)  [unwired: 13 in]
          }
          frame "Macro: Stop Listener" {
            n109 = Unbundle By Name(w324) -> ("SelfRef"=w323:refnum<class "RemoteControl.lvclass">)
            n110 = call <vilib>:"Get LV Class Name.vi"("error in (no error)"=w321, "object"=w323) -> ("error out"=w320:errorcluster, "class name"=w322:string)  [unwired: 8 in]
            n111 = case shown="\"RemoteControl.STM.lvclass\"" w322 {
              tunnel: ["" ("State(s) in Front (\"\")") "RC: Stop Listener SMO\nRC: Destroy Listener SMO" ("State(s) in Front (\"\")")] -> w325
              frame Default {
              }
              frame "RemoteControl.STM.lvclass" {
              }
            }
            n112 = call <vilib>:"Add State(s) to Queue__jki_lib_state_machine.vi"("State(s) in Front (\"\")"=w325, "State(s) in (\"\")"=w328) -> ("States Out"=w327:string)  [unwired: 13 in]
          }
          frame "Macro: RC Exit" {
            n113 = Unbundle By Name(w332) -> ("RC Process Type"=w331:T4)
            n114 = case shown="\"Server\"" w331 {
              tunnel: ["Listener: Stop Listener" ("State(s) in Front (\"\")") "Macro: Stop Listener\nRC: Close Connection" ("State(s) in Front (\"\")")] -> w333
              frame "Listener", Default {
              }
              frame "Server" {
              }
            }
            n115 = call <vilib>:"Add State(s) to Queue__jki_lib_state_machine.vi"("State(s) in Front (\"\")"=w333, "State(s) in (\"\")"=w337) -> ("States Out"=w336:string)  [unwired: 13 in]
          }
          frame "Macro: Post Error Handler" {
            # "Clear Last Error?"
            n116 = Unbundle By Name(w347) -> ("Core.Last Error.error"=w342:errorcluster)
            n117 = Unbundle By Name(w347) -> ("RC Process Type"=w343:T4, "Core.Last Error.remaining states"=w346:string, "Core.Shutdown?"=w345:bool)
            n118 = case shown="False" FALSE {
              tunnel: w342 -> [w355 _]
              tunnel: [w355 _] -> w340
              frame False {
              }
              frame True {
              }
            }
            n119 = case shown="False" w345 {
              tunnel: w346 -> [_ w361]
              tunnel: [w356 w360] -> w344
              tunnel: w343 -> [w357 _]
              frame False {
                # "These are the remaining states (at the moment the error occured). States can be altered according to business logic."
                # "NOT SHUTTING DOWN"
                n120 = case shown="\"Server\"" w357 {
                  tunnel: ["" ("State(s) in Front (\"\")") "Macro: RC Exit\nMacro: RC Initialize" ("State(s) in Front (\"\")")] -> w356
                  frame Default {
                    # "If Listener, owner will restart\nListener process"
                  }
                  frame "Server" {
                  }
                }
              }
              frame True {
                # "Developer can decide to alter the states but should be aware that during the shutdown process, there are certain states that must be run for the SMO to properly shut itself (and this process) down. As such, one can add states to perform additional clean-ups, but should append the remaining state to be executed."
                # "SHUTTING DOWN"
                n121 = call <vilib>:"Add State(s) to Queue__jki_lib_state_machine.vi"("State(s) in (\"\")"=w361) -> ("States Out"=w360:string)  [unwired: 14 in]
              }
            }
            n122 = Bundle By Name(cluster=w347, "Core.Last Error.error"=w340, "Messages (out)"=T3[] [], "state"=enum16{"waiting", "processing"}."waiting") -> (w350:T7)
            n123 = call <vilib>:"Add State(s) to Queue__jki_lib_state_machine.vi"("State(s) in Front (\"\")"=w344, "State(s) in (\"\")"=w354) -> ("States Out"=w353:string)  [unwired: 13 in]
          }
          frame "Macro: Exit" {
            # "Exit Macro\n(This is called once, when the VI exits)"
            n124 = Unbundle By Name(w364) -> ("Core.Close Panel on Exit?"=w366:bool)
            n125 = Bundle By Name(cluster=w364, "Core.Shutdown?"=TRUE) -> (w365:T7)
            n126 = Select(t="UI: Front Panel State >> Close", s=w366, f="") -> (s? t:f=w372:string)
            n127 = call <vilib>:"Add State(s) to Queue__jki_lib_state_machine.vi"("State(s) in Front (\"\")"="Macro: RC Exit", "State(s) at Back (\"\")"="Data: Cleanup\nEvents: Unregister\nProcess: Sync\nExit") -> ("States Out"=w367:string)  [unwired: 13 in]
            n128 = call <vilib>:"Add State(s) to Queue__jki_lib_state_machine.vi"("State(s) in (\"\")"=w372, "State(s) at Back (\"\")"=w367) -> ("States Out"=w371:string)  [unwired: 13 in]
            n129 = call <vilib>:"Add State(s) to Queue__jki_lib_state_machine.vi"("State(s) in Front (\"\")"=w371, "State(s) in (\"\")"=w376) -> ("States Out"=w375:string)  [unwired: 13 in]
          }
          frame "---------- Process ----------" {
            # "Template Separator\n(You can make a copy of, or modify, this frame)"
            n130 = call <vilib>:"Add State(s) to Queue__jki_lib_state_machine.vi"("State(s) in (\"\")"=w381) -> ("States Out"=w380:string)  [unwired: 14 in]
          }
          frame "Process: Sync" {
            n131 = Unbundle By Name(w389) -> ("SelfRef"=w382:refnum<class "RemoteControl.lvclass">)
            n132 = call <vilib>:"WaitOnProcessSync.vi"("error in (no error)"=w385, "SMO"=w382) -> ("error out"=w384:errorcluster, "Don't run?"=w388:bool)  [unwired: 7 in, 1 out]
            n133 = Select(t="Data: Cleanup\nEvents: Unregister\nExit", s=w388, f="") -> (s? t:f=w383:string)
            n134 = call <vilib>:"Add State(s) to Queue__jki_lib_state_machine.vi"("State(s) in Front (\"\")"=w383, "State(s) in (\"\")"=w392) -> ("States Out"=w391:string)  [unwired: 13 in]
          }
          frame "Process: SelfTerminate" {
            n135 = Unbundle By Name(w393) -> ("SelfRef"=w397:refnum<class "RemoteControl.lvclass">)
            n136 = call <vilib>:"SelfTerminate.vi"("error in (no error)"=w395, "SMO in"=w397) -> ("error out"=w394:errorcluster, "SMO out"=w396:refnum<class "RemoteControl.lvclass">)  [unwired: 8 in]
            n137 = Bundle By Name(cluster=w393, "SelfRef"=w396) -> (w398:T7)
            n138 = call <vilib>:"Add State(s) to Queue__jki_lib_state_machine.vi"("State(s) in (\"\")"=w401) -> ("States Out"=w400:string)  [unwired: 14 in]
          }
          frame "---------- Events ----------" {
            # "Template Separator\n(You can make a copy of, or modify, this frame)"
            n139 = call <vilib>:"Add State(s) to Queue__jki_lib_state_machine.vi"("State(s) in (\"\")"=w406) -> ("States Out"=w405:string)  [unwired: 14 in]
          }
          frame "Events: Register" {
            w408 = T10 {"Error"=refnum, "State"=refnum, "Reserve State"=refnum}  # Listener Public Events
            # "Expand to add\nmore events"
            n140 = Unbundle By Name(w418) -> ("SelfRef"=w407:refnum<class "RemoteControl.lvclass">)
            n141 = call <vilib>:"GetProtectedEvents.vi"("SMO"=w407) -> ("error out"=w412:errorcluster, "SMO Protected Events"=w416:T11, "SMO out"=w410:refnum<class "RemoteControl.lvclass">)  [unwired: 8 in]
            n142 = call "RemoteControl.GetPrivateEvents.vi"("RemoteControl"=w410) -> ("error out"=w411:errorcluster, "RC Private Events"=w409:T12)  [unwired: 8 in, 1 out]
            n143 = register-events(w416, w409, w408) -> (reference out=w417:refnum<event-registration>, error out=w413:errorcluster)  [unwired: 2 in]
            n144 = Merge Errors(w411, w415, w413, w412) -> (w414:errorcluster)
            n145 = call <vilib>:"Add State(s) to Queue__jki_lib_state_machine.vi"("State(s) in (\"\")"=w420) -> ("States Out"=w419:string)  [unwired: 14 in]
          }
          frame "Events: Register Listener SMO" {
            w425 = T10 {"Error"=refnum, "State"=refnum, "Reserve State"=refnum}  # Listener Public Events
            n146 = Unbundle By Name(w432) -> ("Listener"=w426:refnum<class "RemoteControl.lvclass">)
            n147 = call <vilib>:"GetPublicEvents.vi"("SMO"=w426) -> ("error out"=w424:errorcluster, "Public Events"=w422:T10)  [unwired: 8 in, 1 out]
            n148 = Variant To Data(error in=w424, type=w425, Variant=w422) -> (data=w421:T10, error out=w423:errorcluster)
            n149 = register-events(reference=w427, w421) -> (reference out=w431:refnum<event-registration>, error out=w428:errorcluster)  [unwired: 3 in]
            n150 = Merge Errors(w430, w428, w423) -> (w429:errorcluster)
            n151 = call <vilib>:"Add State(s) to Queue__jki_lib_state_machine.vi"("State(s) in (\"\")"=w434) -> ("States Out"=w433:string)  [unwired: 14 in]
          }
          frame "Events: Unregister" {
            n152 = Unregister For Events(event registration refnum=w437, error in=w436) -> (error out=w435:errorcluster)
            n153 = call <vilib>:"Clear Errors.vi"("error in (no error)"=w435) -> ()  [unwired: 5 in, 2 out]
            n154 = call <vilib>:"Add State(s) to Queue__jki_lib_state_machine.vi"("State(s) in (\"\")"=w440) -> ("States Out"=w439:string)  [unwired: 14 in]
          }
          frame "---------- RC ----------" {
            # "Template Separator\n(You can make a copy of, or modify, this frame)"
            n155 = call <vilib>:"Add State(s) to Queue__jki_lib_state_machine.vi"("State(s) in (\"\")"=w445) -> ("States Out"=w444:string)  [unwired: 14 in]
          }
          frame "RC: Send Messages to Owner" {
            # "This loop will run # times equal to messages in the queue"
            # "Send Message to Owner to be processed\n(Send a message to the instrument to be processed)"
            n156 = Unbundle By Name(w446) -> ("SelfRef"=w450:refnum<class "RemoteControl.lvclass">, "Messages (in)"=w447:T3[])
            n157 = for {
              tunnel: w450 -> [w456]
              tunnel: w449 -> [w460]
              tunnel: w447 -> [w455] mode=indexing
              tunnel: w448 -> [w459]
              tunnel: [w462] -> w451
              n158 = call "Time Message Events.vi"("error in (no error)"=w459, "Debug Mode"=w460, "Message in"=w455, "RemoteControl"=w456) -> ("error out"=w461:errorcluster, "Message out"=w458:T3, "RemoteControl out"=w457:refnum<class "RemoteControl.lvclass">)  [unwired: 4 in, 1 out]
              n159 = call "RemoteControl.SendMessageFromProcess.vi"("error in (no error)"=w461, "Message"=w458, "RemoteControl"=w457) -> ("error out"=w462:errorcluster)  [unwired: 7 in, 1 out]
            }
            n160 = call <vilib>:"Add State(s) to Queue__jki_lib_state_machine.vi"("State(s) in (\"\")"=w454) -> ("States Out"=w453:string)  [unwired: 14 in]
          }
          frame "RC: Get Connections" {
            # "Here listen for new connections and then stop after timeout or if there's a new connection"
            n161 = Unbundle By Name(w471) -> ("SelfRef"=w470:refnum<class "RemoteControl.lvclass">)
            n162 = call-dynamic "Get Connections.vi"("error in (no error)"=w469, "RemoteControl in"=w470) -> ("error out"=w464:errorcluster, "Number"=w467:i32, "RemoteControl out"=w468:refnum<class "RemoteControl.lvclass">)  [unwired: 7 in]
            "Connections" <- w467
            n163 = case shown="Default" w467 {
              selector: w467 -> [_ w482 _]
              tunnel: ["" ("State(s) in Front (\"\")") w481 "RC: Close Connection" ("State(s) in Front (\"\")")] -> w466
              frame 0 {
              }
              frame Default {
                # "read %d messages"
                n164 = Format Into String(format string="RC: Read Messages >> %d" ("State(s) in Front (\"\")"), w482) -> (resulting string=w481:string)  [unwired: 2 in, 1 out]
              }
              frame 100 {
              }
            }
            n165 = Bundle By Name(cluster=w471, "SelfRef"=w468) -> (w472:T7)
            n166 = xnode "Error Ring"() -> ()  [unwired: 1 out]
            n167 = case shown="True" "create server error" {
              tunnel: w464 -> [w477 _]
              tunnel: [w477 errorcluster {"status"=TRUE, "code"=-1001, "source"="Server error"} ("t")] -> w463
              frame False {
              }
              frame True {
                n168 = local write "create server error"(FALSE ("create listener error")) -> ()
              }
            }
            n169 = call <vilib>:"Add State(s) to Queue__jki_lib_state_machine.vi"("State(s) in Front (\"\")"=w466, "State(s) in (\"\")"=w475) -> ("States Out"=w474:string)  [unwired: 13 in]
          }
          frame "RC: Read Messages" {
            # "poll the number\nof open connections"
            # "Read Message over, eg TCP"
            # "If command is empty do not Send Message"
            n170 = Unbundle By Name(w492) -> ("SelfRef"=w491:refnum<class "RemoteControl.lvclass">)
            n171 = Unbundle By Name(w492) -> ("to"=w498:i32)
            n172 = call "Write Timeout.vi"("error in (no error)"=w490, "timeout (ms) [500]"="timeout (ms) [500]", "RemoteControl in"=w491) -> ("error out"=w489:errorcluster, "RemoteControl out"=w488:refnum<class "RemoteControl.lvclass">)  [unwired: 7 in]
            n173 = call-dynamic "Read Message.vi"("error in (no error)"=w489, "RemoteControl in"=w488) -> ("error out"=w496:errorcluster, "Data"=w493:string, "Command"=w494:string, "RemoteControl out"=w495:refnum<class "RemoteControl.lvclass">, "ID"=w497:string)  [unwired: 5 in]
            n174 = case shown="Default" w494 {
              selector: w494 -> [w512 _]
              tunnel: w497 -> [w515 _]
              tunnel: w496 -> [w517 w528]
              tunnel: [w517 w528] -> w500
              tunnel: w505 -> [_ _]
              tunnel: w495 -> [w513 w522]
              tunnel: w493 -> [w516 _]
              tunnel: [enum16{"waiting", "processing"}."processing" ("state") w527] -> w502
              tunnel: enum16{"waiting", "processing"}."waiting" ("state") -> [_ w527]
              tunnel: ["RC: Send Messages to Owner" ""] -> w501
              tunnel: [5000 w526] -> w499
              tunnel: w498 -> [_ w526]
              tunnel: [w514 w523] -> w486
              tunnel: [w513 w522] -> w485
              frame Default {
                n175 = To Variant(anything=w516) -> (Variant=w511:variant)
                n176 = Bundle By Name(cluster=T3 {"Command"="", "Data"=variant(string ""), "ID"=""} ("Message from Remote"), "Command"=w512, "Data"=w511, "ID"=w515) -> (w509:T3)
                n177 = call "Message to Display String.vi"("Message"=w509) -> ("message string"=→"Message In":string)
                n178 = Build Array(w509) -> (w514:T3[])
              }
              frame "" {
                # "Messages coming from TCP need to have command"
                n179 = Build Array(T3 {"Command"="", "Data"=variant(string ""), "ID"=""} ("Message out")) -> (w523:T3[])
              }
            }
            n180 = Bundle By Name(cluster=w492, "to"=w499, "state"=w502, "SelfRef"=w485, "Messages (in)"=w486) -> (w504:T7)
            n181 = call <vilib>:"Add State(s) to Queue__jki_lib_state_machine.vi"("State(s) in Front (\"\")"=w501, "State(s) in (\"\")"=w508) -> ("States Out"=w507:string)  [unwired: 13 in]
          }
          frame "RC: Write Messages" {
            # "After the loop completes\nempty the out queue"
            # "This loop will run # times equal to messages in the out queue"
            # "send Message over, eg. TCP"
            n182 = Unbundle By Name(w534) -> ("SelfRef"=w539:refnum<class "RemoteControl.lvclass">, "Messages (out)"=w537:T3[])
            n183 = for {
              tunnel: w539 -> [w554]
              tunnel: w538 -> [w543]
              tunnel: w537 -> [w544] mode=indexing
              tunnel: [w546] -> w529
              tunnel: w536 -> [w552]
              tunnel: [w553] -> w535
              n184 = call "Time Message Events.vi"("error in (no error)"=w552, "Debug Mode"=w543, "Message in"=w544) -> ("error out"=w551:errorcluster, "Message out"=w545:T3)  [unwired: 5 in, 2 out]
              n185 = Unbundle By Name(w545) -> ("Command"=w547:string, "Data"=w548:variant, "ID"=w549:string)
              n186 = while {
                tunnel: w551 -> [w556]
                tunnel: [w556] -> w550
                stop <- "delay response" continue-if-true
              }
              n187 = call-dynamic "Send Message.vi"("ID"=w549, "error in (no error)"=w550, "Data"=w548, "Command"=w547, "RemoteControl in"=w554) -> ("error out"=w553:errorcluster, "RemoteControl out"=w546:refnum<class "RemoteControl.lvclass">)  [unwired: 5 in]
            }
            n188 = Bundle By Name(cluster=w534, "Messages (out)"=T3[] [], "state"=enum16{"waiting", "processing"}."waiting", "to"=5, "SelfRef"=w529) -> (w533:T7)
            n189 = call <vilib>:"Add State(s) to Queue__jki_lib_state_machine.vi"("State(s) in (\"\")"=w542) -> ("States Out"=w541:string)  [unwired: 14 in]
          }
          frame "RC: Close Connection" {
            # "Closes open server connections"
            # "call this on error 66, etc (when connection\ndrops). check these in error handler"
            n190 = Unbundle By Name(w561) -> ("SelfRef"=w562:refnum<class "RemoteControl.lvclass">)
            n191 = call-dynamic "Close Connection.vi"("error in (no error)"=w558, "RemoteControl in"=w562) -> ("error out"=w557:errorcluster, "RemoteControl out"=w559:refnum<class "RemoteControl.lvclass">)  [unwired: 8 in]
            n192 = Bundle By Name(cluster=w561, "SelfRef"=w559) -> (w560:T7)
            n193 = call <vilib>:"Add State(s) to Queue__jki_lib_state_machine.vi"("State(s) in (\"\")"=w565) -> ("States Out"=w564:string)  [unwired: 14 in]
          }
          frame "RC: Create Listener SMO" {
            # "Create Listener SMO"
            n194 = Unbundle By Name(w575) -> ("SelfRef"=w568:refnum<class "RemoteControl.lvclass">, "Configure"=w570:T6)
            n195 = Bundle By Name(cluster=w568, "Configure"=w570, "RC Process Type"=RC_Process_Type--Enum."Listener") -> (w567:refnum<class "RemoteControl.lvclass">)
            n196 = call <vilib>:"Create.vi"("error in (no error)"=w566, "Subsystem Name (optional)"="Remote-Control-Listener" ("format string"), "SMO"=w567) -> ("error out"=w573:errorcluster, "SMO out"=w569:refnum<class "RemoteControl.lvclass">)  [unwired: 6 in, 1 out]
            n197 = Bundle By Name(cluster=w575, "Listener"=w569) -> (w574:T7)
            n198 = call <vilib>:"Add State(s) to Queue__jki_lib_state_machine.vi"("State(s) in (\"\")"=w578) -> ("States Out"=w577:string)  [unwired: 14 in]
          }
          frame "RC: Start Listener SMO" {
            n199 = Unbundle By Name(w584) -> ("Listener"=w581:refnum<class "RemoteControl.lvclass">)
            n200 = call <vilib>:"Start.vi"("error in (no error)"=w580, "SMO"=w581) -> ("error out"=w579:errorcluster, "SMO out"=w582:refnum<class "RemoteControl.lvclass">)  [unwired: 8 in]
            n201 = Bundle By Name(cluster=w584, "Listener"=w582) -> (w583:T7)
            n202 = call <vilib>:"Add State(s) to Queue__jki_lib_state_machine.vi"("State(s) in (\"\")"=w587) -> ("States Out"=w586:string)  [unwired: 14 in]
          }
          frame "RC: Stop Listener SMO" {
            n203 = Unbundle By Name(w591) -> ("Listener"=w592:refnum<class "RemoteControl.lvclass">)
            n204 = call <vilib>:"Stop.vi"("error in (no error)"=w589, "SMO"=w592) -> ("error out"=w588:errorcluster, "SMO out"=w593:refnum<class "RemoteControl.lvclass">)  [unwired: 8 in]
            n205 = Bundle By Name(cluster=w591, "Listener"=w593) -> (w590:T7)
            n206 = call <vilib>:"Add State(s) to Queue__jki_lib_state_machine.vi"("State(s) in (\"\")"=w596) -> ("States Out"=w595:string)  [unwired: 14 in]
          }
          frame "RC: Destroy Listener SMO" {
            n207 = Unbundle By Name(w597) -> ("Listener"=w598:refnum<class "RemoteControl.lvclass">)
            n208 = call <vilib>:"Destroy.vi"("error in (no error)"=w600, "SMO"=w598) -> ("error out"=w599:errorcluster)  [unwired: 9 in]
            n209 = call <vilib>:"Add State(s) to Queue__jki_lib_state_machine.vi"("State(s) in (\"\")"=w603) -> ("States Out"=w602:string)  [unwired: 14 in]
          }
          frame "RC: Open Client Connection" {
            n210 = Unbundle By Name(w607) -> ("SelfRef"=w611:refnum<class "RemoteControl.lvclass">, "Configure.address"=w605:string, "Configure.Port"=w604:u16)
            n211 = call-dynamic "Open Client Connection.vi"("error in (no error)"=w610, "Port"=w604, "address"=w605, "RemoteControl in"=w611) -> ("error out"=w609:errorcluster, "RemoteControl out"=w608:refnum<class "RemoteControl.lvclass">)  [unwired: 6 in]
            n212 = Bundle By Name(cluster=w607, "SelfRef"=w608) -> (w606:T7)
            n213 = call <vilib>:"Add State(s) to Queue__jki_lib_state_machine.vi"("State(s) in (\"\")"=w614) -> ("States Out"=w613:string)  [unwired: 14 in]
          }
          frame "RC: Open Server Connection" {
            n214 = Unbundle By Name(w618) -> ("SelfRef"=w622:refnum<class "RemoteControl.lvclass">, "Configure.address"=w616:string, "Configure.Port"=w615:u16)
            n215 = call-dynamic "Open Server Connection.vi"("error in (no error)"=w621, "Port"=w615, "address"=w616, "RemoteControl in"=w622) -> ("error out"=w620:errorcluster, "RemoteControl out"=w619:refnum<class "RemoteControl.lvclass">)  [unwired: 6 in]
            n216 = Bundle By Name(cluster=w618, "SelfRef"=w619) -> (w617:T7)
            n217 = call <vilib>:"Add State(s) to Queue__jki_lib_state_machine.vi"("State(s) in (\"\")"=w625) -> ("States Out"=w624:string)  [unwired: 14 in]
          }
          frame "---------- Listener ----------" {
            # "Template Separator\n(You can make a copy of, or modify, this frame)"
            n218 = call <vilib>:"Add State(s) to Queue__jki_lib_state_machine.vi"("State(s) in (\"\")"=w630) -> ("States Out"=w629:string)  [unwired: 14 in]
          }
          frame "Listener: Start Listener" {
            # "Start Asynchronous Listener"
            n219 = Unbundle By Name(w631) -> ("SelfRef"=w636:refnum<class "RemoteControl.lvclass">)
            n220 = call-dynamic "Start Listener.vi"("error in (no error)"=w635, "RemoteControl in"=w636) -> ("error out"=w634:errorcluster, "RemoteControl out"=w633:refnum<class "RemoteControl.lvclass">)  [unwired: 8 in]
            n221 = Bundle By Name(cluster=w631, "SelfRef"=w633) -> (w632:T7)
            n222 = call <vilib>:"Add State(s) to Queue__jki_lib_state_machine.vi"("State(s) in (\"\")"=w639) -> ("States Out"=w638:string)  [unwired: 14 in]
          }
          frame "Listener: Listen" {
            n223 = Unbundle By Name(w648) -> ("SelfRef"=w645:refnum<class "RemoteControl.lvclass">)
            n224 = call-dynamic "Listen.vi"("timeout ms (100) (wait forever: -1)"=1000, "error in (no error)"=w644, "RemoteControl"=w645) -> ("error out"=w641:errorcluster, "RemoteControl out"=w646:refnum<class "RemoteControl.lvclass">)  [unwired: 7 in]
            n225 = Bundle By Name(cluster=w648, "SelfRef"=w646) -> (w647:T7)
            n226 = case shown="True" "create listener error" {
              tunnel: w641 -> [w652 _]
              tunnel: [w652 errorcluster {"status"=TRUE, "code"=-1000, "source"="Listener error"} ("t")] -> w640
              frame False {
              }
              frame True {
                n227 = local write "create listener error"(FALSE ("create listener error")) -> ()
              }
            }
            n228 = call <vilib>:"Add State(s) to Queue__jki_lib_state_machine.vi"("State(s) in (\"\")"=w651) -> ("States Out"=w650:string)  [unwired: 14 in]
          }
          frame "Listener: Stop Listener" {
            # "Stop Asynchronous Listener \n(You can make a copy of, or modify, this frame)"
            n229 = Unbundle By Name(w655) -> ("SelfRef"=w658:refnum<class "RemoteControl.lvclass">)
            n230 = call-dynamic "Stop Listener.vi"("error in (no error)"=w657, "RemoteControl in"=w658) -> ("error out"=w656:errorcluster)  [unwired: 8 in, 1 out]
            n231 = call <vilib>:"Add State(s) to Queue__jki_lib_state_machine.vi"("State(s) in (\"\")"=w661) -> ("States Out"=w660:string)  [unwired: 14 in]
          }
        }
      }
    }
    frame Error {
    }
  }
  n232 = call-parent "Process.vi"("error in"=w3, "SMO"=w2) -> ("error out"=w1:errorcluster, "SMO out"=→"RemoteControl out":refnum<class "RemoteControl.lvclass">)  [unwired: 8 in]
  n233 = Merge Errors(w1, w5) -> (→"error out":errorcluster)
